vi "NewTemplate.Init.vi"(6 "JQMHStartup in":refnum<class "RQMHStartup.lvclass">, 8 "error in (no error)":errorcluster, 11 "NewTemplate in":refnum<class "NewTemplate.lvclass">) -> (0 "error out":errorcluster, 1 "StartupParams":variant, 2 "Requests":T2, 3 "NewTemplate out":refnum<class "NewTemplate.lvclass">, 4 "JQMHStartup out":refnum<class "RQMHStartup.lvclass">, 5 "StandardRequests":refnum<event-registration>)   [LabVIEW 2024, in "NewTemplate.lvclass"]
uses:
  NewTemplate.lvclass
  C:/DevOps/CORTEX/JQMH/JQMHCore/Module/RQMHModule.lvclass
  JQMHCore/JQMHStartup/RQMHStartup.lvclass
  JQMHCore/Module/StopEventArgs.ctl
  Request Events--cluster.ctl
  Do Something Args.ctl
  JQMHCore/Module/Reply.ctl
  JQMHCore/Module/StandardRequests.ctl
  JQMHCore/Module/InitialiseArgs.ctl
  JQMHCore/Module/Show Front Panel--Args.ctl
  JQMHCore/Module/Hide Front Panel.ctl
  JQMHCore/Module/Show Block Diagram.ctl
  JQMHCore/Module/Hide Block Diagram--Args.ctl
  JQMHCore/Module/RQMHModule.lvclass/RQMHModule.ctl
  NewTemplate.lvclass/NewTemplate.ctl
  JQMHCore/Shared/JQMHShared.lvlib
  JQMHCore/Module/RQMHModule.lvclass
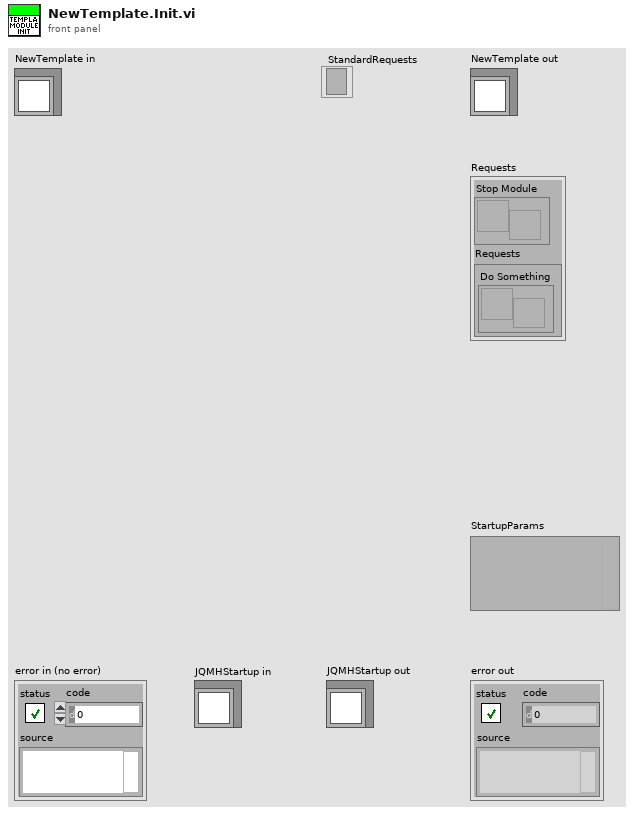
[diagram p1: front panel]
types:
  T1 = typedef "NewTemplate.lvclass/Request Events--cluster.ctl" = cluster{"Do Something":refnum<user-event>}
  T2 = cluster{"Stop Module":refnum<user-event>, "Requests":T1}
  T3 = typedef "RQMHModule.lvclass/StandardRequests.ctl" = cluster{"Initialise":refnum<user-event>, "Stop Module":refnum<user-event>, "ShowFP":refnum<user-event>, "Hide Front Panel":refnum<user-event>, "Show Block Diagram":refnum<user-event>, "Hide Block Diagram":refnum<user-event>}
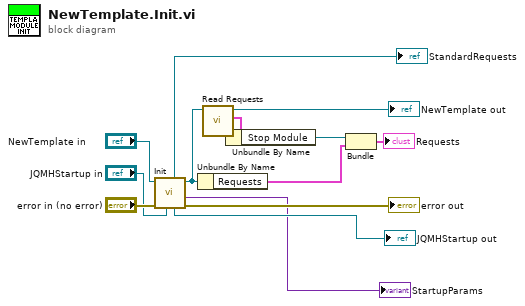
[diagram p0: block diagram]
diagram:
  n1 = call "Init.vi"("JQMHStartup.lvclass"="JQMHStartup in", "error in (no error)"="error in (no error)", "JQMHCore.lvclass"="NewTemplate in") -> ("error out"=→"error out":errorcluster, "StartupParams"=→"StartupParams":variant, "JQMHCore out"=w12:refnum<class "NewTemplate.lvclass">, "JQMHStartup out"=→"JQMHStartup out":refnum<class "RQMHStartup.lvclass">, "Event Registration Refnum"=→"StandardRequests":refnum<event-registration>)  [unwired: 4 in]
  n2 = Unbundle By Name(w12) -> ("Requests"=w13:T1)
  n3 = call "Read Requests.vi"("JQMHModule in"=w12) -> ("Requests"=w5:T3, "JQMHModule out"=→"NewTemplate out":refnum<class "NewTemplate.lvclass">)  [unwired: 9 in]
  n4 = Unbundle By Name(w5) -> ("Stop Module"=w4:refnum<user-event>)
  n5 = Bundle("Stop Module"=w4, "Requests"=w13) -> (→"Requests":T2)  [unwired: 1 in]
